vi "save auto coag data.vi"(9 "averaged data":T1 {"DOM coag demand (mg/L)" min=0.0 max=200.0; "Coag dose (mg/L)" min=0.1 max=200.0}) -> ()   [LabVIEW 2019]
uses:
  data cluster.ctl
  file paths.ctl
panel:
  out "data labels":string[](array[string])
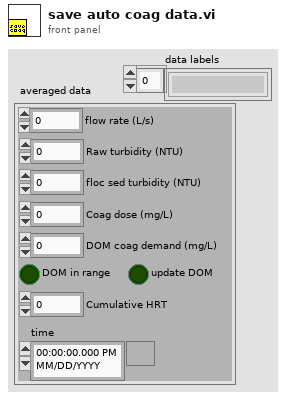
[diagram p1: front panel]
types:
  T1 = typedef "data cluster.ctl" = cluster{"floc sed turbidity (NTU)":dbl, "Raw turbidity (NTU)":dbl, "flow rate (L/s)":dbl, "time":timestamp, "Cumulative HRT":dbl, "Coag dose (mg/L)":dbl, "DOM coag demand (mg/L)":dbl, "DOM in range":bool, "update DOM":bool}
  T2 = typedef "file paths.ctl" = enum16{"read paths", "close"}
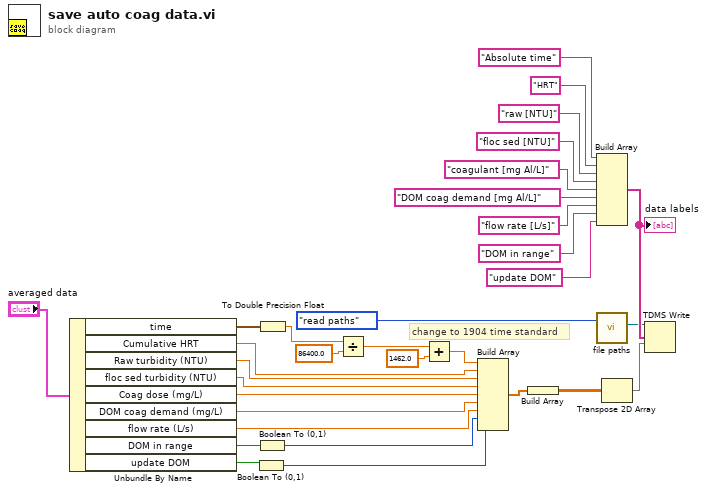
[diagram p0: block diagram]
diagram:
  # "change to 1904 time standard"
  n1 = Unbundle By Name("averaged data") -> ("time"=w13:timestamp, "Cumulative HRT"=w11:dbl, "Raw turbidity (NTU)"=w10:dbl, "floc sed turbidity (NTU)"=w9:dbl, "Coag dose (mg/L)"=w8:dbl, "DOM coag demand (mg/L)"=w7:dbl, "flow rate (L/s)"=w6:dbl, "DOM in range"=w12:bool, "update DOM"=w3:bool)
  n2 = Boolean To (0,1)(Boolean=w3) -> (0, 1=w2:i16)
  n3 = Boolean To (0,1)(Boolean=w12) -> (0, 1=w27:i16)
  n4 = To Double Precision Float(number=w13) -> (double precision float=w23:dbl)
  n5 = Divide(x=w23, y=86400.0) -> (x/y=w21:dbl)
  n6 = Add(x=w21, y=1462.0) -> (x+y=w19:dbl)
  n7 = Build Array(w19, w11, w10, w9, w8, w7, w6, w27, w2) -> (w26:dbl[])
  n8 = Build Array(w26) -> (w25:dbl[][])
  n9 = Build Array("Absolute time", "HRT", "raw [NTU]", "floc sed [NTU]", "coagulant [mg Al/L]" ("element"), "DOM coag demand [mg Al/L]" ("element"), "flow rate [L/s]" ("element"), "DOM in range" ("element"), "update DOM" ("element")) -> (w28:string[])
  "data labels" <- w28
  n10 = call "file paths.vi"("file path control"=file_paths."read paths") -> ("coaglog"=w14:refnum<k34>)  [unwired: 7 in, 3 out]
  n11 = Transpose 2D Array(2D array=w25) -> (transposed array=w24:dbl[][])
  n12 = TDMS Write(0:w14, 7:w28, 9:w24) -> ()  [unwired: 3 in, 4 out]
